vi "Mensaje_1.vi"(0 "cancelled":bool, 5 "Error In":errorcluster) -> (19 "Error Out":errorcluster)   [LabVIEW 2013]
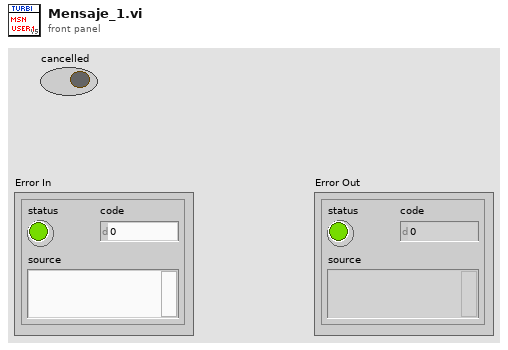
[diagram p1: front panel]
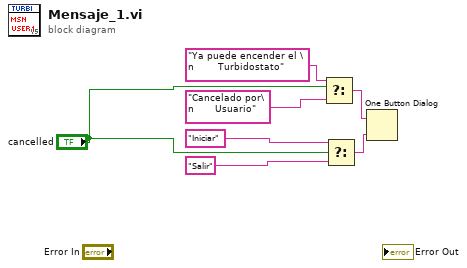
[diagram p0: block diagram]
diagram:
  n1 = Select(t="Ya puede encender el \n        Turbidostato" ("message"), s="cancelled", f="Cancelado por\n       Usuario" ("message")) -> (s? t:f=w4:string)
  n2 = Select(t="Iniciar" ("button name (\"OK\")"), s="cancelled", f="Salir" ("button name (\"OK\")")) -> (s? t:f=w1:string)
  n3 = One Button Dialog(message=w4, button name ("OK")=w1) -> ()  [unwired: 1 out]
